vi "TDMS Saver.vi"(10 "TDMS Cluster":T1, 11 "Data to Log":dbl[](array[numeric])) -> ()   [LabVIEW 2014]
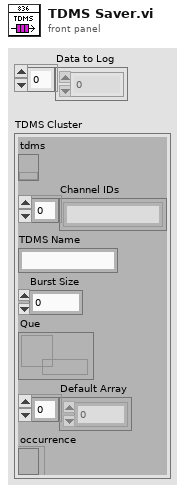
[diagram p1: front panel]
types:
  T1 = cluster{"tdms":refnum<k34>, "Channel IDs":string[], "TDMS Name":string, "Burst Size":i32, "Que":refnum<k33>, "Default Array":dbl[], "occurrence":refnum<k4>}
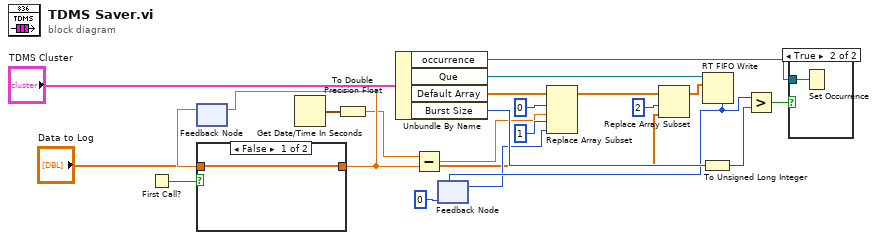
[diagram p0: block diagram]
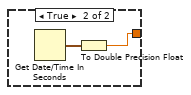
[diagram p2: hidden frame]
diagram:
  n1 = First Call?() -> (First Call?: T/F=w14:bool)
  n2 = feedback #1() -> (w15:dbl)  [unwired: 1 in]
  n3 = case shown="False" w14 {
    tunnel: [w23 w24] -> w16
    tunnel: w15 -> [w23 _]
    frame False {
    }
    frame True {
      n4 = Get Date/Time In Seconds() -> (seconds since 1Jan1904=w25:timestamp)
      n5 = To Double Precision Float(number=w25) -> (double precision float=w24:dbl)
    }
  }
  n6 = feedback-in #1(w16) -> ()
  n7 = Get Date/Time In Seconds() -> (seconds since 1Jan1904=w2:timestamp)
  n8 = To Double Precision Float(number=w2) -> (double precision float=w3:dbl)
  n9 = Unbundle By Name("TDMS Cluster") -> ("occurrence"=w18:refnum<k4>, "Que"=w20:refnum<k33>, "Default Array"=w19:dbl[], "Burst Size"=w21:i32)
  n10 = Subtract(x=w3, y=w16) -> (x-y=w4:dbl)
  n11 = feedback #2(u32 0 ("# elements")) -> (w10:u32)
  n12 = Replace Array Subset(array=w19, new element #1=w4, index #1=0 ("index"), new element #2=w10, index #2=1 ("index")) -> (w5:dbl[])
  n13 = Replace Array Subset(array=w5, new element="Data to Log", index=2) -> (w8:dbl[])
  n14 = To Unsigned Long Integer(number=w21) -> (unsigned 32bit integer=w22:u32)
  n15 = RT FIFO Write(0:w20, 1:w8) -> (7:w12:u32)  [unwired: 3 in, 3 out]
  n16 = feedback-in #2(w12) -> ()
  n17 = Greater?(x=w12, y=w22) -> (0:w13:bool)
  n18 = case shown="True" w13 {
    tunnel: w18 -> [_ w26]
    frame False {
    }
    frame True {
      n19 = Set Occurrence(w26) -> ()
    }
  }
